vi "EPTx-RT-Loop.vi"() -> ()   [LabVIEW 2019]
uses:
  <vilib>/Platform/TimedLoop/XDataNode/XDataNode.xnode
  <vilib>/Platform/TimedLoop/XDataNode/nitl_modes.ctl
  <vilib>/Platform/TimedLoop/XDataNode/XDNodeRunTimeDep.lvlib
  <vilib>/Platform/TimedLoop/XDataNode/wakeup.ctl
  <vilib>/Platform/TimedLoop/XDataNode/timing_clust.ctl
  <vilib>/rvi/interface/nirviReadWriteControl/nirviReadWriteControl.xnode
  <vilib>/rvi/interface/Simulation/niFpgaSimulationCallBeginRW.vi
  <vilib>/rvi/errors/niLvFpgaAdjustHostInterfaceError.vi
  <vilib>/rvi/interface/nirviOpenFPGA/nirviOpenFPGA.xnode
  <vilib>/Powertrain Controls/Device Drivers/Engine Position Tracking/EPTx/RevA/RT/EPTx - RevA - RT.lvlib
  <vilib>/Utility/error.llb/Error Cluster From Error Code.vi
  NiFpgaLv.dll
  <vilib>/rvi/interface/nirviCloseFPGA/nirviCloseFPGA.xnode
  <vilib>/FPGAPlugInAG/Dynamic/niLvFpga_Close_Dynamic.vi
  FPGA/EPTx FPGA-Loop.vi
  <vilib>/userDefined/High Color/nirio_resource_hc.ctl
  <vilib>/Powertrain Controls/Device Drivers/Engine Position Tracking/EPTx/RevA/RT/Controls/EPTxState.ctl
  <vilib>/Powertrain Controls/Device Drivers/Engine Position Tracking/EPTx/RevA/RT/Controls/EPTxFilters.ctl
  <vilib>/Powertrain Controls/Device Drivers/Engine Position Tracking/EPTx/RevA/RT/Controls/EPTxAAPControl.ctl
  <vilib>/Powertrain Controls/Device Drivers/Engine Position Tracking/EPTx/RevA/RT/Controls/EPTxData.ctl
  <vilib>/Powertrain Controls/Device Drivers/Engine Position Tracking/EPTx/RevA/RT/Controls/Pattern Config.ctl
  <vilib>/Powertrain Controls/Device Drivers/Engine Position Tracking/EPTx/RevA/RT/Controls/Simulator Config.ctl
panel:
  in  "Pattern Filename":string="YC-6kcfg.EPTxP"
  out "EPTxDebug":T1
  out "Pattern Loading":bool
  out "Sim Loading":bool
  in  "SimulatorConfig":T2={"Sim Speed [RPM]"=1000.0, "Ramp Rate [RPM/s]"=50.0, "Rotations"=2, "Pause"=FALSE, "Pause Angle [CAD]"=0.0, "Max Offset [RPM]"=0.0, "Cylinders"=6}
  in  "PatternConfig":T3 {"Max Rate [Hz]" format="%#_3p"}
  in  "Load":bool
  out "EPTxData":T4
  out "循环持续时间":i64
  out "Config Loading":bool
  out "错误输出":errorcluster
  in  "CamSim_AAPControl":T5
  in  "History (63) [CAD]":u8=63
  in  "Filters (0)":T6={"Primary [s]"=5e-06, "Aux 1 [s]"=5e-06, "Aux 2 [s]"=0.0, "Aux 3 [s]"=0.0, "Aux 4 [s]"=0.0} {"Aux 4 [s]" format="%#_6p"; "Aux 3 [s]" format="%#_6p"; "Aux 2 [s]" format="%#_6p"; "Aux 1 [s]" format="%#_6p"; "Primary [s]" format="%#_6p"}
  in  "Stall Speed (200) [RPM]":sgl=200.0
  in  "EPTxState":T7
  in  "Configuration Filename":string="YC-6kcfg.EPTx"
  in  "资源名称":T8="PXI1Slot7" caption="RIO设备"
  # "Clear error不建议为true，否则将无法识别错误"
  # "模拟Supervisor，忽略外部位置信号，根据转速模拟Supervisor position"
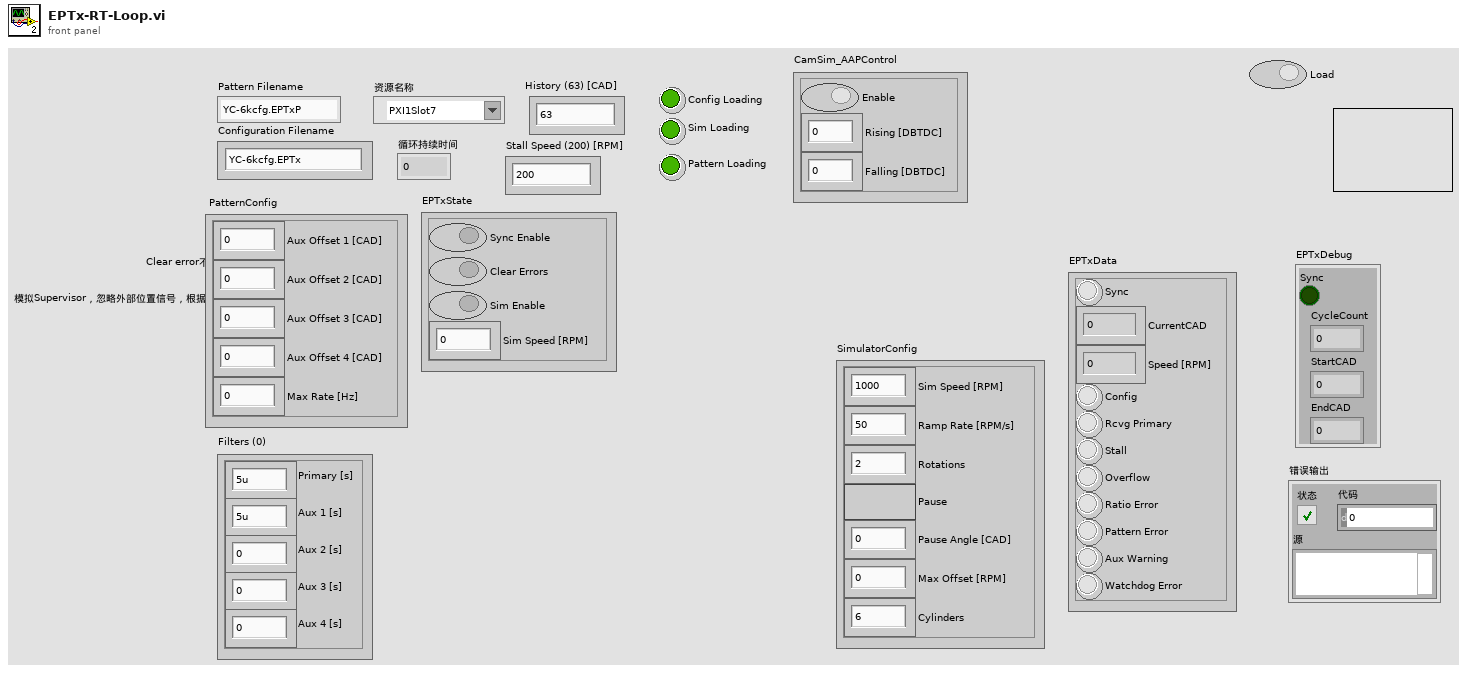
[diagram p1: front panel]
types:
  T1 = cluster{"Sync":bool, "CycleCount":fxp<+,8,8>, "StartCAD":fxp<+,18,11>, "EndCAD":fxp<+,18,11>}
  T2 = typedef "EPTx - RevA - RT.lvlib/Simulator Config.ctl" = cluster{"Sim Speed [RPM]":sgl, "Ramp Rate [RPM/s]":sgl, "Rotations":u8, "Pause":bool, "Pause Angle [CAD]":sgl, "Max Offset [RPM]":sgl, "Cylinders":u8}
  T3 = typedef "EPTx - RevA - RT.lvlib/Pattern Config.ctl" = cluster{"Aux Offset 1 [CAD]":sgl, "Aux Offset 2 [CAD]":sgl, "Aux Offset 3 [CAD]":sgl, "Aux Offset 4 [CAD]":sgl, "Max Rate [Hz]":sgl}
  T4 = typedef "EPTx - RevA - RT.lvlib/EPTxData.ctl" = cluster{"Sync":bool, "CurrentCAD":sgl, "Speed [RPM]":sgl, "Config":bool, "Rcvg Primary":bool, "Stall":bool, "Overflow":bool, "Ratio Error":bool, "Pattern Error":bool, "Aux Warning":bool, "Watchdog Error":bool}
  T5 = typedef "EPTx - RevA - RT.lvlib/EPTxAAPControl.ctl" = cluster{"Enable":bool, "Rising [DBTDC]":sgl, "Falling [DBTDC]":sgl}
  T6 = typedef "EPTx - RevA - RT.lvlib/EPTxFilters.ctl" = cluster{"Primary [s]":sgl, "Aux 1 [s]":sgl, "Aux 2 [s]":sgl, "Aux 3 [s]":sgl, "Aux 4 [s]":sgl}
  T7 = typedef "EPTx - RevA - RT.lvlib/EPTxState.ctl" = cluster{"Sync Enable":bool, "Clear Errors":bool, "Sim Enable":bool, "Sim Speed [RPM]":sgl}
  T8 = typedef "nirio_resource_hc.ctl" = tag
  T9 = typedef "XDNodeRunTimeDep.lvlib/timing_clust.ctl" = cluster{"Expected End [f-1]":u64, "Actual End [f-1]":u64, "Finished Late? [f-1]":bool, "Expected End [i-1]":u64, "Actual End [i-1]":u64, "Finished Late? [i-1]":bool, "Expected Start [i]":u64, "Actual Start [i]":u64, "Expected Start [f]":u64, "Actual Start [f]":u64, "Source Name":string, "Structure Name":string, "Period":i64, "Deadline":i64, "Offset":i64, "Start":i64, "Priority":i32, "Timeout":i32, "Mode":T10, "Wakeup Reason":T11, "Error":errorcluster, "Source Type":string, "Secondary Source Type":string, "Global End Time":u64, "Global Start Time":u64, "Frame Duration":u64, "Iteration Duration":u64, "Assigned CPU":i32, "I/O Scan Engine Mode":u32}
  T10 = typedef "XDNodeRunTimeDep.lvlib/nitl_modes.ctl" = enum32{"No Change", "Process missed periods, maintain original phase", "Discard missed periods, maintain original phase", "Process missed periods, ignore original phase", "Discard missed periods, ignore original phase"}
  T11 = typedef "XDNodeRunTimeDep.lvlib/wakeup.ctl" = enum32{"Normal", "Aborted", "Asynchronous wakeup", "Timing source error", "Timed loop error", "Timeout"}
  T12 = cluster{"Sync":bool, "CurrentCAD":fxp<+,18,11>, "MaxCAD":fxp<+,11,11>, "HistoryCAD":fxp<+,11,11>, "CADRate":fxp<+,22,8>, "AvgSpeed":fxp<+,17,15>, "Config":bool, "Rcvg Primary":bool, "Stall":bool, "Overflow":bool, "Ratio Error":bool, "Pattern Error":bool, "Aux Warning":bool, "Watchdog Error":bool}
  T13 = typedef "EPTx - RevA - RT.lvlib/EPTxSettings.ctl" = cluster{"Rotation":u8, "Ratios":sgl[], "Thresholds":sgl[], "Tooth":T14, "Pattern":T16[], "Token":T17[], "Aux Threshold Min":T20, "Aux Threshold Max":T20}
  T14 = typedef "EPTx - RevA - RT.lvlib/Settings - Tooth.ctl" = cluster{"Rising Edge":bool, "Falling Edge":bool, "Direction\nDetection":T15, "Level":bool, "Parameter":sgl}
  T15 = typedef "EPTx - RevA - RT.lvlib/Direction Detection.ctl" = enum16{"None", "Aux Signal", "Length"}
  T16 = typedef "EPTx - RevA - RT.lvlib/Settings - Pattern.ctl" = cluster{"Ratio Index":u8, "Ratio Count":u16, "Angle":sgl, "dAngle":sgl}
  T17 = typedef "EPTx - RevA - RT.lvlib/Settings - Token.ctl" = cluster{"Length":u16, "Start Index":u8, "Start Count":u16, "Aux 1":T18, "Aux 1 Type":T19, "Aux 1 Max":u16, "Aux 1 Min":u16, "Aux 2":T18, "Aux 2 Type":T19, "Aux 2 Max":u16, "Aux 2 Min":u16, "End Index":u8, "End Count":u16}
  T18 = typedef "EPTx - RevA - RT.lvlib/Aux Signal.ctl" = enum8{"---", "Aux 1", "Aux 2", "Aux 3", "Aux 4"}
  T19 = typedef "EPTx - RevA - RT.lvlib/Aux Type.ctl" = enum8{"Falling", "Rising", "Low", "High", "Ratio"}
  T20 = typedef "EPTx - RevA - RT.lvlib/Aux Threshold.ctl" = cluster{"Aux 1":sgl, "Aux 2":sgl, "Aux 3":sgl, "Aux 4":sgl}
  T21 = typedef "EPTx - RevA - FPGA.lvlib/EPTxConfig.ctl" = u64
  T22 = typedef "EPTx - RevA - FPGA.lvlib/EPTxControl.ctl" = cluster{"Sync Enable":bool, "Clear Errors":bool, "Sim Enable":bool, "Sim Rate":fxp<+,24,6>, "Watchdog":bool}
  T23 = typedef "EPTx - RevA - FPGA.lvlib/EPTxSimulatorConfig.ctl" = u32
  T24 = typedef "EPTx - RevA - RT.lvlib/EPTxPattern.ctl" = cluster{"Rotations":u8, "Cylinders":u8, "Primary":T25[], "Aux 1":T25[], "Aux 2":T25[], "Aux 3":T25[], "Aux 4":T25[]}
  T25 = typedef "EPTx - RevA - RT.lvlib/Pattern.ctl" = cluster{"Angle":sgl, "State":bool}
  T26 = typedef "EPTx - RevA - FPGA.lvlib/EPTxPatternConfig.ctl" = cluster{"Address":fxp<+,14,14>, "Pattern":T27}
  T27 = typedef "EPTx - RevA - FPGA.lvlib/Patterns.ctl" = cluster{"Primary":fxp<+,19,12>, "Primary State":bool, "Aux 1":fxp<+,19,12>, "Aux 1 State":bool, "Aux 2":fxp<+,19,12>, "Aux 2 State":bool, "Aux 3":fxp<+,19,12>, "Aux 3 State":bool, "Aux 4":fxp<+,19,12>, "Aux 4 State":bool}
  T28 = typedef "EPTx - RevA - FPGA.lvlib/EPTxAAPControl.ctl" = cluster{"Enable":bool, "RisingCAD":fxp<+,18,11>, "FallingCAD":fxp<+,18,11>}
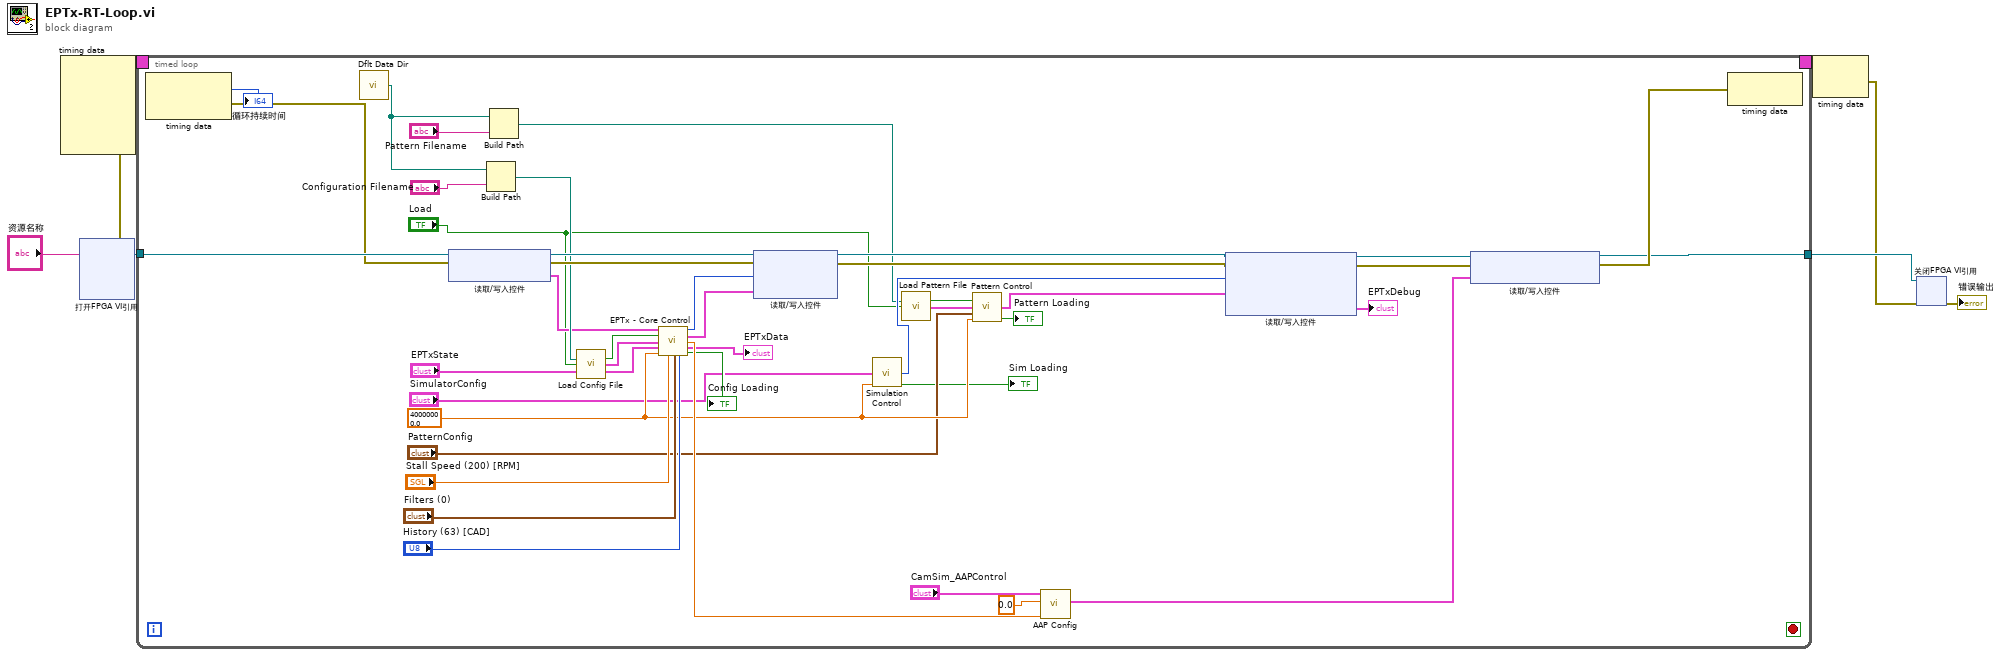
[diagram p0: block diagram]
diagram:
  n1 = xnode "打开FPGA VI引用"("资源名称"="资源名称") -> ("FPGA VI引用输出"=w4:refnum<k20>, "错误输出"=w5:errorcluster)  [unwired: 1 in]
  n2 = node-c288(w5) -> (w8:T9)  [unwired: 4 in]
  n3 = timed-loop {
    timing: w8 -> [_]
    timing-out: [_] -> w7
    tunnel: w4 -> [w50]
    tunnel: [w32] -> w3
    stop <- _ stop-if-true
    w24 = sgl 40000000.0 ("Frequency (40M) [Hz]")
    n4 = node-c288() -> (→"循环持续时间":i64, w49:errorcluster)  [unwired: 1 in]
    n5 = call <vilib>:"Dflt Data Dir.vi"() -> ("App:Default Data Directory"=w11:path)
    n6 = xnode "读取/写入控件"("FPGA VI引用输入"=w50, "错误输入"=w49) -> ("FPGA VI引用输出"=w48:refnum<k20>, "错误输出"=w47:errorcluster, "EPTxSupervisor"=w30:T12)
    n7 = Build Path(base path=w11, name or relative path="Configuration Filename") -> (appended path=w45:path)
    n8 = Build Path(base path=w11, name or relative path="Pattern Filename") -> (appended path=w12:path)
    n9 = call <vilib>:"Load Config File.vi"("Configuration Path"=w45, "Load"="Load") -> ("Loaded"=w43:bool, "EPTxSettings"=w44:T13)  [unwired: 12 in]
    n10 = call <vilib>:"EPTx - Core Control.vi"("EPTxSupervisor"=w30, "Load"=w43, "EPTxSettings"=w44, "EPTxState"="EPTxState", "Frequency (40M) [Hz]"=w24, "Stall Speed (200) [RPM]"="Stall Speed (200) [RPM]", "Filters (0)"="Filters (0)", "History (63) [CAD]"="History (63) [CAD]") -> ("EPTxConfig"=w38:T21, "EPTxControl"=w37:T22, "Max CAD"=w34:sgl, "EPTxData"=→"EPTxData":T4, "Loading"=→"Config Loading":bool)  [unwired: 3 in]
    n11 = xnode "读取/写入控件"("FPGA VI引用输入"=w48, "错误输入"=w47, "EPTxConfig"=w38, "EPTxControl"=w37) -> ("FPGA VI引用输出"=w19:refnum<k20>, "错误输出"=w18:errorcluster)
    n12 = call <vilib>:"Simulation Control.vi"("SimulatorConfig"="SimulatorConfig", "Frequency (40M) [Hz]"=w24) -> ("EPTxSimulatorConfig"=w14:T23, "Loading"=→"Sim Loading":bool)  [unwired: 12 in]
    n13 = call <vilib>:"Load Pattern File.vi"("Pattern Path"=w12, "Load"="Load") -> ("Loaded"=w26:bool, "EPTxPatternSettings"=w25:T24)  [unwired: 12 in]
    n14 = call <vilib>:"Pattern Control.vi"("Load"=w26, "EPTxPatternSettings"=w25, "PatternConfig"="PatternConfig", "Frequency (40M) [Hz]"=w24) -> ("EPTxPatternConfig"=w9:T26, "Loading"=→"Pattern Loading":bool)  [unwired: 10 in]
    n15 = call <vilib>:"AAP Config.vi"("Max CAD"=w34, "Cylinder TDC [Absolute CAD]"=sgl 0.0, "EPTxAAPControl"="CamSim_AAPControl") -> ("EPTxAAPControl"=w35:T28)  [unwired: 8 in]
    n16 = xnode "读取/写入控件"("FPGA VI引用输入"=w19, "错误输入"=w18, "EPTxSimulatorConfig"=w14, "EPTxPatternConfig"=w9) -> ("FPGA VI引用输出"=w16:refnum<k20>, "错误输出"=w17:errorcluster, "EPTxDebug"=→"EPTxDebug":T1)
    n17 = xnode "读取/写入控件"("FPGA VI引用输入"=w16, "错误输入"=w17, "CamSim_AAPControl"=w35) -> ("FPGA VI引用输出"=w32:refnum<k20>, "错误输出"=w33:errorcluster)
    n18 = node-c288(w33) -> ()  [unwired: 1 out]
  }
  n19 = node-c288(w7) -> (w2:errorcluster)
  n20 = xnode "关闭FPGA VI引用"("FPGA VI引用输入"=w3, "错误输入"=w2) -> ("错误输出"=→"错误输出":errorcluster)
